vi "Generate Nonce.vi"() -> (3 "Noce":string)   [LabVIEW 2020, in "wamplv.lvlib" / "WampScramAuthenticator.lvclass"]
uses:
  WampScramAuthenticator.lvclass
  <vilib>/numeric/Random Number (Range) U64.vi
  <vilib>/numeric/sub_Random U32.vi
  Utils/Base64 Encode.vi
  Utils/Utils.lvclass
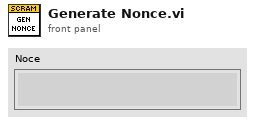
[diagram p1: front panel]
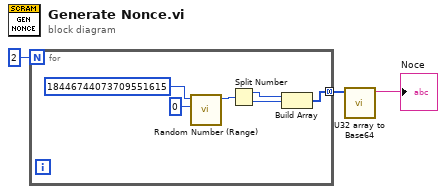
[diagram p0: block diagram]
diagram:
  n1 = for {
    N: 2 -> [_]
    tunnel: [w4] -> w2 mode=concatenating
    n2 = call-poly <vilib>:"Random Number (Range).vi"("lower bound (0)"=u64 0, "upper bound (100)"=u64 18446744073709551615) -> ("number"=w7:u64)  [unwired: 9 in]
    n3 = Split Number(x=w7) -> (hi(x)=w6:u32, lo(x)=w5:u32)
    n4 = Build Array(w6, w5) -> (w4:u32[])
  }
  n5 = call "U32 array to Base64.vi"("Array"=w2) -> ("Base64 sring out"=→"Noce":string)  [unwired: 10 in]
